vi "Nimbelink_Database_Ops_No_SQL_Open_Close.vi"(0 "Operation":T1(ring)=enum."Get Col Names", 1 "Find column":u16(ring) items=["work_order", "btw_sn", "mac", "meid", "operator", "datetime", "part_number", "imei", "sim_id", "phone", "test_result"], 2 "table name":string="test_data", 5 "Record data":string[](array[string])=["wo12345", "123450001", "70B3D55A8100", "A1001234567890", "Joe", "2013-05-07 10:28:19", "100013", "353123456789012", "89123456789012345678", "612-555-1212", "Pass", "", "", "", "", "", "", "", "", "", "", "", "", "", "", "", "", "", "", "", "", "", "", "", "", "", "", "", "", "", "", "", "", "", "", "", "", "", "", "", "", "", "", "", "", "", "", "", "", "", "", "", "12:01:00"], 7 "Connection In":refnum<k7>, 9 "SQL Query":string="Insert into dbo.test_data VALUES ", 11 "Error in (no error)":errorcluster, 12 "Find data":string, 13 "Insert fields":i32=23) -> (3 "Found?":bool, 4 "RecordSet":string[][](array[string]), 6 "Column Names":string[](array[string])=["work_order", "btw_sn", "mac", "meid", "operator", "date_time", "part_number", "imei", "sim_id", "phone_number", "test_result", "board_sn", "test_time", "test_program", "test_version", "extra1", "extra2", "guid", "extra3", "extra4", "extra5", "extra6", "extra7"], 8 "Connection Out":refnum<k7>, 10 "Records":i32, 14 "Last test passed?":bool, 15 "Error out":errorcluster)   [LabVIEW 2013]
panel:
  out "Find return string":string
  out "Final query string":string="select column_name,* from information_schema.columns\n where table_name = 'test_data'\norder by ordinal_position"
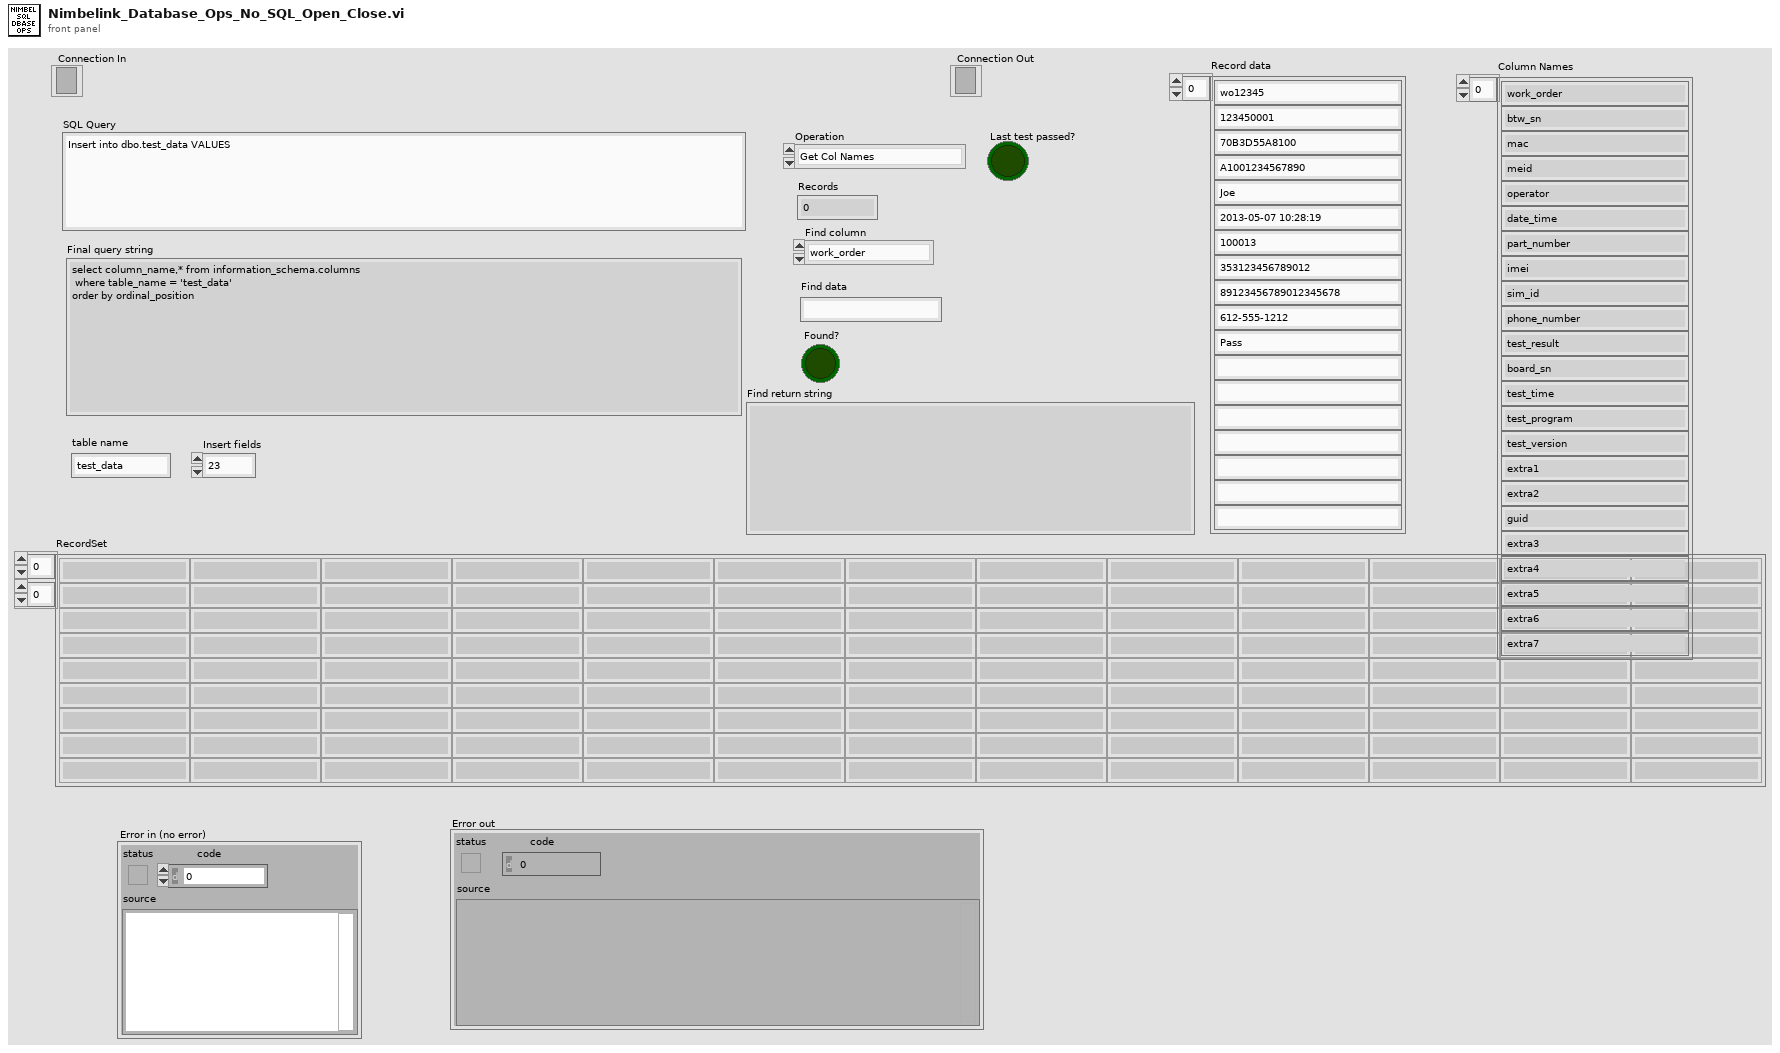
[diagram p1: front panel]
types:
  T1 = enum16{"Query", "Insert", "Select", "Dump Recs", "Get Rec Count", "Get Col Names", "Insert all fields", "Find", "Get last test result", "Get work order qty", "Set work order qty", "Save test report", "Get test report", "Execute query no data", "Select count", "Query and return row 0 col 0"}
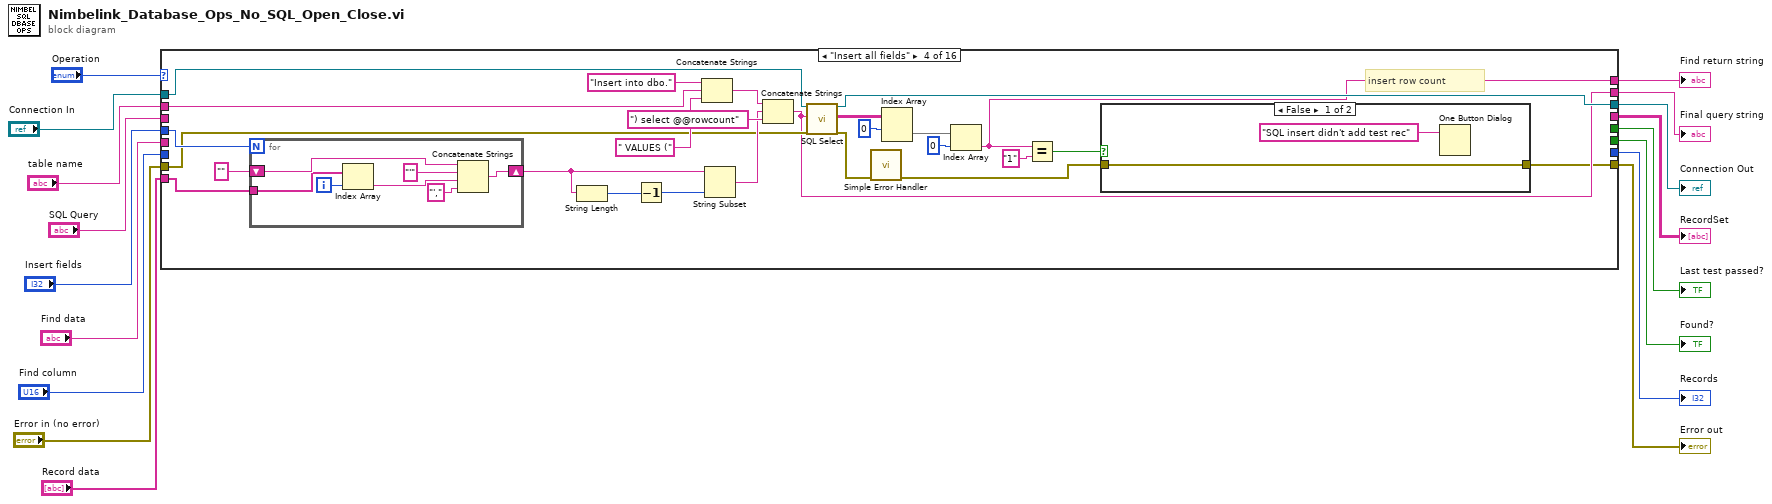
[diagram p0: block diagram]
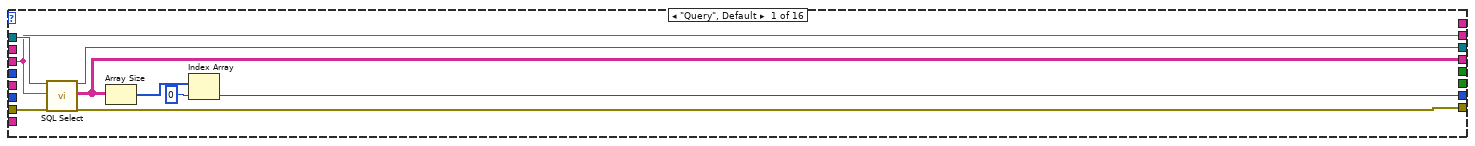
[diagram p2: hidden frame]
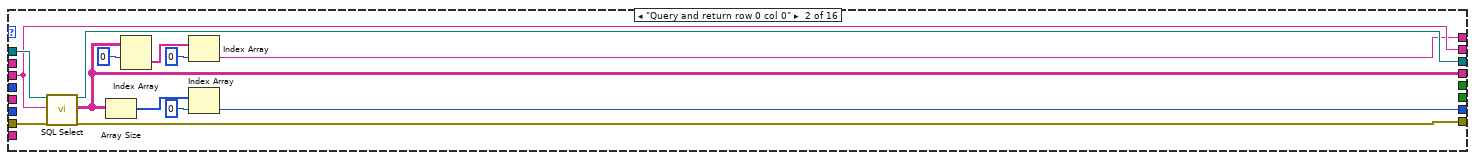
[diagram p3: hidden frame]
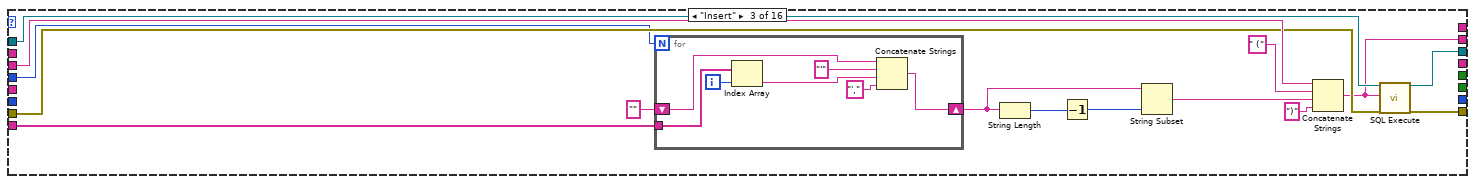
[diagram p4: hidden frame]
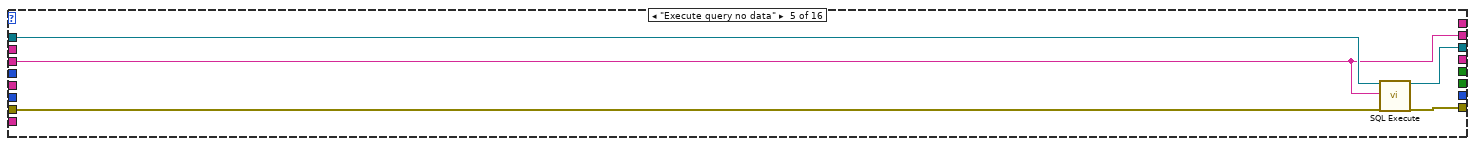
[diagram p6: hidden frame]
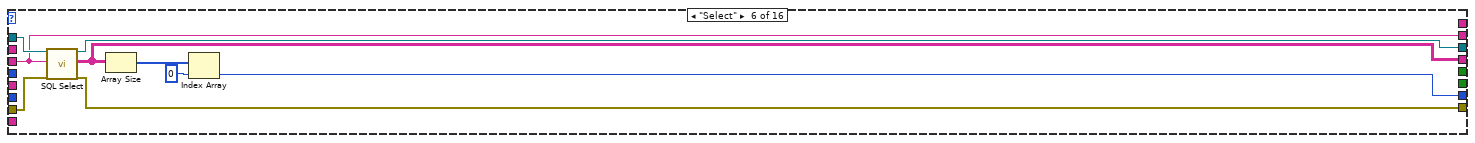
[diagram p7: hidden frame]
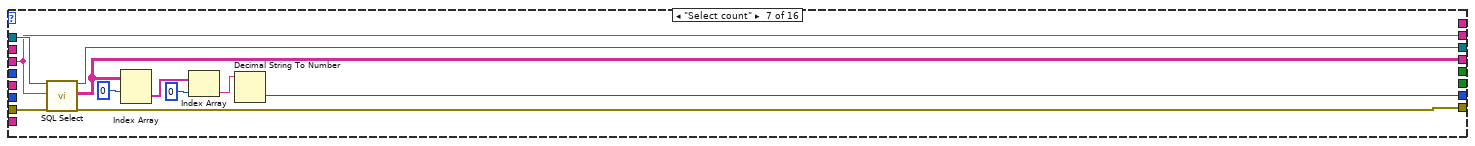
[diagram p8: hidden frame]
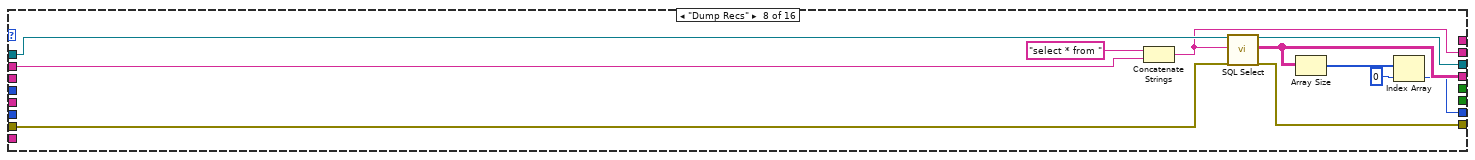
[diagram p9: hidden frame]
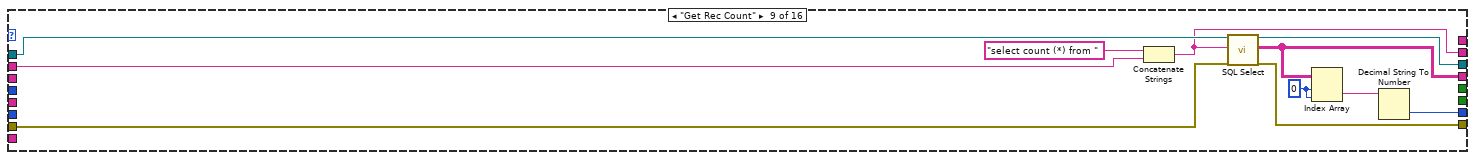
[diagram p10: hidden frame]
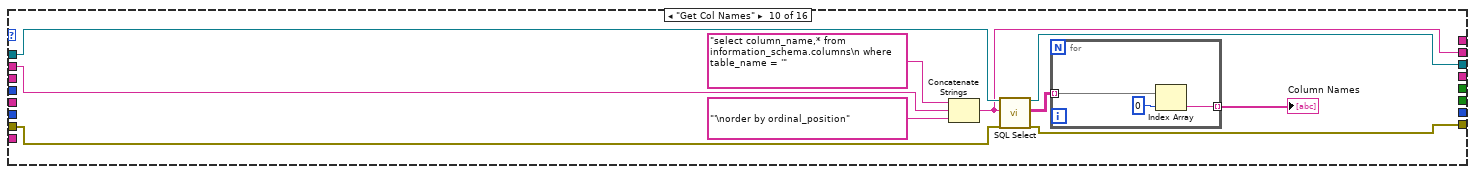
[diagram p11: hidden frame]
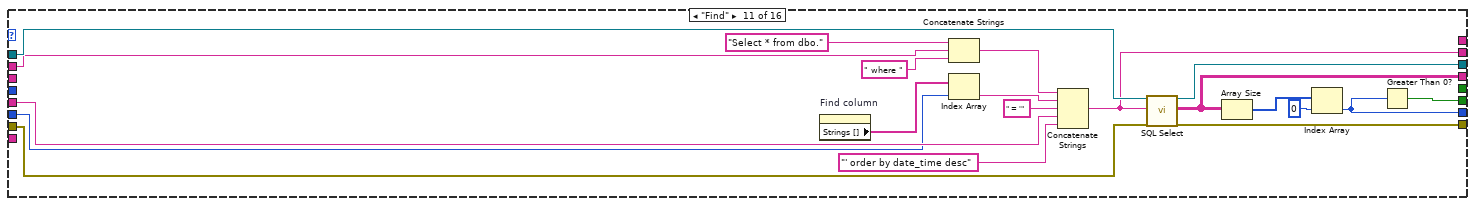
[diagram p12: hidden frame]
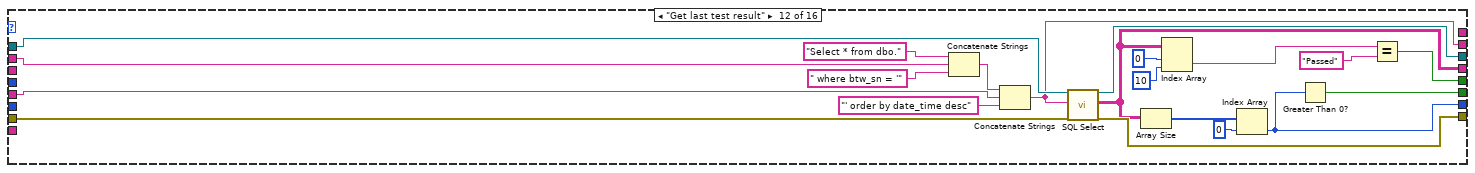
[diagram p13: hidden frame]
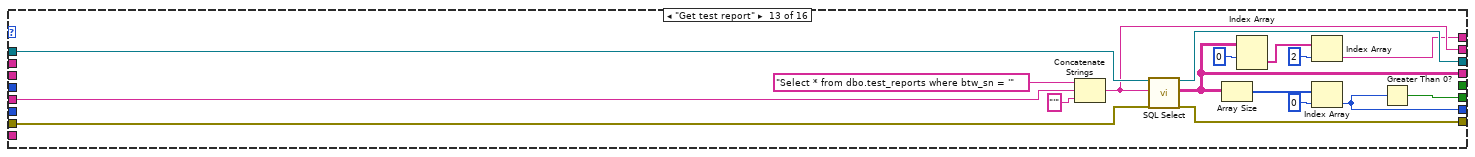
[diagram p14: hidden frame]
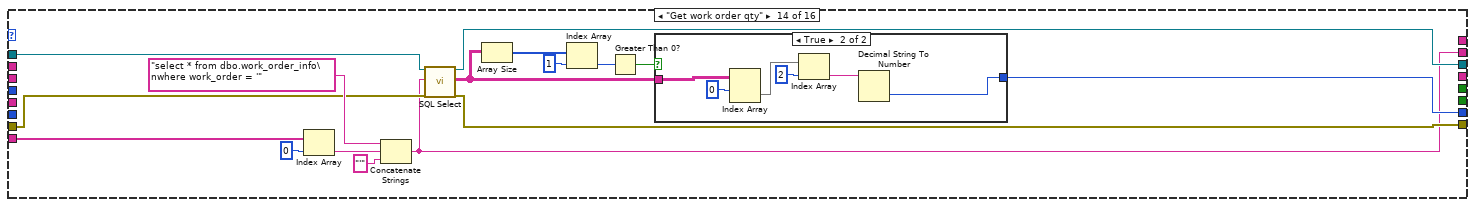
[diagram p15: hidden frame]
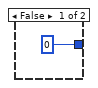
[diagram p16: hidden frame]
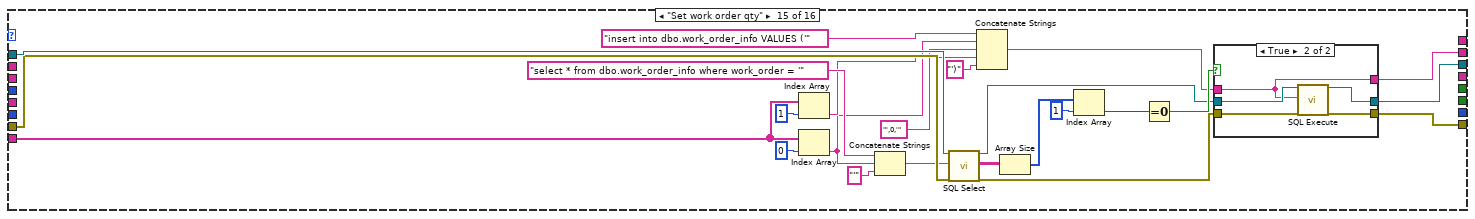
[diagram p17: hidden frame]
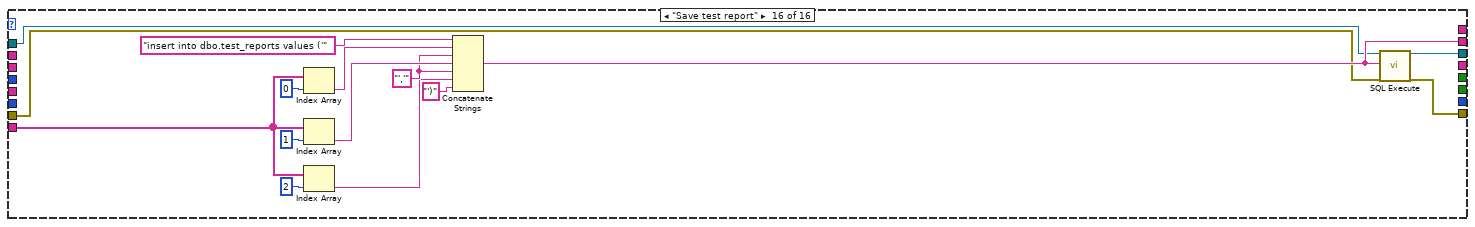
[diagram p19: hidden frame]
diagram:
  n1 = case shown="\"Insert all fields\"" "Operation" {
    tunnel: [w25 w38 w54 w62 w102 w108 w119 w130 w141 w150 w171 w195 w212 w220 w246 w280] -> w1
    tunnel: [w23 w36 w53 w74 w101 w109 w120 w131 w142 w149 w173 w197 w214 w222 w245 w279] -> w17
    tunnel: "Connection In" -> [w24 w37 w52 w75 w100 w110 w121 w133 w144 w154 w174 w198 w215 w223 w262 w276]
    tunnel: "Error in (no error)" -> [w26 w39 w42 w73 w99 w111 w122 w132 w143 w153 w172 w196 w213 w225 w259 w277]
    tunnel: "SQL Query" -> [w22 w35 w47 _ w98 w107 w118 _ _ _ _ _ _ _ _ _]
    tunnel: [w19 w31 _ _ _ w104 w117 w126 w136 _ w168 w183 w203 _ _ _] -> w12
    tunnel: "Record data" -> [_ _ w51 w87 _ _ _ _ _ _ _ _ _ w224 w251 w275]
    tunnel: [w22 w35 w41 w68 w98 w107 w118 w129 w138 w148 w167 w192 w209 w219 w244 w278] -> w13
    tunnel: "table name" -> [_ _ _ w80 _ _ _ w128 w139 w146 w164 w189 _ _ _ _]
    tunnel: [w18 w32 _ _ _ w103 w112 w123 w135 _ w161 w186 w207 w221 _ _] -> w10
    tunnel: [_ _ _ _ _ _ _ _ _ _ w160 w185 w206 _ _ _] -> w9
    tunnel: "Find data" -> [_ _ _ _ _ _ _ _ _ _ w159 w184 w205 _ _ _]
    tunnel: "Find column" -> [_ _ _ _ _ _ _ _ _ _ w158 _ _ _ _ _]
    tunnel: [_ _ _ _ _ _ _ _ _ _ _ w178 _ _ _ _] -> w6
    tunnel: "Insert fields" -> [_ _ w40 w76 _ _ _ _ _ _ _ _ _ _ _ _]
    tunnel: [_ w27 _ w66 _ _ _ _ _ _ _ _ w200 _ _ _] -> w4
    frame "Query", Default {
      n2 = call "SQL Select.vi"("Connection In"=w24, "SQL Query"=w22, "Error in (no error)"=w26) -> ("Connection Out"=w23:refnum<k7>, "Data"=w19:string[][], "Error out"=w25:errorcluster)  [unwired: 14 in]
      n3 = Array Size(array=w19) -> (size(s)=w21:i32[])
      n4 = Index Array(array=w21, index=0) -> (element=w18:i32)
    }
    frame "Query and return row 0 col 0" {
      n5 = call "SQL Select.vi"("Connection In"=w37, "SQL Query"=w35, "Error in (no error)"=w39) -> ("Connection Out"=w36:refnum<k7>, "Data"=w31:string[][], "Error out"=w38:errorcluster)  [unwired: 14 in]
      n6 = Array Size(array=w31) -> (size(s)=w34:i32[])
      n7 = Index Array(array=w31, index (row)=0) -> (element=w29:string[])  [unwired: 1 in]
      n8 = Index Array(array=w29, index=0) -> (element=w27:string)
      n9 = Index Array(array=w34, index=0) -> (element=w32:i32)
    }
    frame "Insert" {
      n10 = for {
        N: w40 -> [_]
        tunnel: w51 -> [w57]
        shift-right: [w60] -> w44
        shift-left: "" -> [w59]
        i -> [w56]
        n11 = Index Array(array=w57, index=w56) -> (element=w55:string)
        n12 = Concatenate Strings(w59, "'" ("string"), w55, "'," ("string")) -> (w60:string)
      }
      n13 = String Length(string=w44) -> (length=w46:i32)
      n14 = Decrement(x=w46) -> (x-1=w45:i32)
      n15 = String Subset(string=w44, length (rest)=w45) -> (substring=w43:string)  [unwired: 1 in]
      n16 = Concatenate Strings(w47, " (" ("string"), w43, ")") -> (w41:string)
      n17 = call "SQL Execute.vi"("Connection In"=w52, "SQL Query"=w41, "Error in (no error)"=w42) -> ("Connection Out"=w53:refnum<k7>, "Error out"=w54:errorcluster)  [unwired: 15 in]
    }
    frame "Insert all fields" {
      # "insert row count"
      n18 = for {
        N: w76 -> [_]
        tunnel: w87 -> [w93]
        shift-right: [w96] -> w82
        shift-left: "" -> [w95]
        i -> [w92]
        n19 = Index Array(array=w93, index=w92) -> (element=w91:string)
        n20 = Concatenate Strings(w95, "'" ("string"), w91, "'," ("string")) -> (w96:string)
      }
      n21 = String Length(string=w82) -> (length=w84:i32)
      n22 = Decrement(x=w84) -> (x-1=w83:i32)
      n23 = Concatenate Strings("Insert into dbo." ("string"), w80, " VALUES (" ("string")) -> (w79:string)
      n24 = String Subset(string=w82, length (rest)=w83) -> (substring=w81:string)  [unwired: 1 in]
      n25 = Concatenate Strings(w79, w81, ") select @@rowcount") -> (w68:string)
      n26 = call "SQL Select.vi"("Connection In"=w75, "SQL Query"=w68, "Error in (no error)"=w73) -> ("Connection Out"=w74:refnum<k7>, "Data"=w69:string[][], "Error out"=w67:errorcluster)  [unwired: 14 in]
      n27 = call <vilib>:"Simple Error Handler.vi"("error in (no error)"=w67) -> ("error out"=w63:errorcluster)  [unwired: 4 in, 4 out]
      n28 = Index Array(array=w69, index (row)=0) -> (element=w71:string[])  [unwired: 1 in]
      n29 = Index Array(array=w71, index=0) -> (element=w66:string)
      n30 = Equal?(x=w66, y="1") -> (x = y?=w64:bool)
      n31 = case shown="False" w64 {
        tunnel: w63 -> [w88 w90]
        tunnel: [w88 w90] -> w62
        frame False {
          n32 = One Button Dialog(message="SQL insert didn't add test rec") -> ()  [unwired: 1 in, 1 out]
        }
        frame True {
        }
      }
    }
    frame "Execute query no data" {
      n33 = call "SQL Execute.vi"("Connection In"=w100, "SQL Query"=w98, "Error in (no error)"=w99) -> ("Connection Out"=w101:refnum<k7>, "Error out"=w102:errorcluster)  [unwired: 15 in]
    }
    frame "Select" {
      n34 = call "SQL Select.vi"("Connection In"=w110, "SQL Query"=w107, "Error in (no error)"=w111) -> ("Connection Out"=w109:refnum<k7>, "Data"=w104:string[][], "Error out"=w108:errorcluster)  [unwired: 14 in]
      n35 = Array Size(array=w104) -> (size(s)=w106:i32[])
      n36 = Index Array(array=w106, index=0) -> (element=w103:i32)
    }
    frame "Select count" {
      n37 = call "SQL Select.vi"("Connection In"=w121, "SQL Query"=w118, "Error in (no error)"=w122) -> ("Connection Out"=w120:refnum<k7>, "Data"=w117:string[][], "Error out"=w119:errorcluster)  [unwired: 14 in]
      n38 = Index Array(array=w117, index (row)=0) -> (element=w115:string[])  [unwired: 1 in]
      n39 = Index Array(array=w115, index=0) -> (element=w113:string)
      n40 = Decimal String To Number(string=w113) -> (number=w112:i32)  [unwired: 2 in, 1 out]
    }
    frame "Dump Recs" {
      n41 = Concatenate Strings("select * from " ("SQL Query"), w128) -> (w129:string)
      n42 = call "SQL Select.vi"("Connection In"=w133, "SQL Query"=w129, "Error in (no error)"=w132) -> ("Connection Out"=w131:refnum<k7>, "Data"=w126:string[][], "Error out"=w130:errorcluster)  [unwired: 14 in]
      n43 = Array Size(array=w126) -> (size(s)=w125:i32[])
      n44 = Index Array(array=w125, index=0) -> (element=w123:i32)
    }
    frame "Get Rec Count" {
      w140 = 0 ("index (row)")
      n45 = Concatenate Strings("select count (*) from " ("SQL Query"), w139) -> (w138:string)
      n46 = call "SQL Select.vi"("Connection In"=w144, "SQL Query"=w138, "Error in (no error)"=w143) -> ("Connection Out"=w142:refnum<k7>, "Data"=w136:string[][], "Error out"=w141:errorcluster)  [unwired: 14 in]
      n47 = Index Array(array=w136, index (row)=w140, index (col)=w140) -> (element=w134:string)
      n48 = Decimal String To Number(string=w134) -> (number=w135:i32)  [unwired: 2 in, 1 out]
    }
    frame "Get Col Names" {
      n49 = Concatenate Strings("select column_name,* from information_schema.columns\n where table_name = '" ("SQL Query"), w146, "'\norder by ordinal_position" ("SQL Query")) -> (w148:string)
      n50 = call "SQL Select.vi"("Connection In"=w154, "SQL Query"=w148, "Error in (no error)"=w153) -> ("Connection Out"=w149:refnum<k7>, "Data"=w152:string[][], "Error out"=w150:errorcluster)  [unwired: 14 in]
      n51 = for {
        tunnel: w152 -> [w157] mode=indexing
        tunnel: [w156] -> w151 mode=indexing
        n52 = Index Array(array=w157, index=0 ("index (col)")) -> (element=w156:string)
      }
      "Column Names" <- w151
    }
    frame "Find" {
      n53 = property on="Find column" class="Ring (strict)"() -> ("Strings []"=w177:string[])  [unwired: 2 in, 2 out]
      n54 = Concatenate Strings("Select * from dbo." ("string"), w164, " where " ("string")) -> (w166:string)
      n55 = Index Array(array=w177, index=w158) -> (element=w176:string)
      n56 = Concatenate Strings(w166, w176, " = '" ("string"), w159, "' order by date_time desc" ("string")) -> (w167:string)
      n57 = call "SQL Select.vi"("Connection In"=w174, "SQL Query"=w167, "Error in (no error)"=w172) -> ("Connection Out"=w173:refnum<k7>, "Data"=w168:string[][], "Error out"=w171:errorcluster)  [unwired: 14 in]
      n58 = Array Size(array=w168) -> (size(s)=w169:i32[])
      n59 = Index Array(array=w169, index=0) -> (element=w161:i32)
      n60 = Greater Than 0?(x=w161) -> (x > 0?=w160:bool)
    }
    frame "Get last test result" {
      n61 = Concatenate Strings("Select * from dbo." ("string"), w189, " where btw_sn = '" ("string")) -> (w191:string)
      n62 = Concatenate Strings(w191, w184, "' order by date_time desc" ("string")) -> (w192:string)
      n63 = call "SQL Select.vi"("Connection In"=w198, "SQL Query"=w192, "Error in (no error)"=w196) -> ("Connection Out"=w197:refnum<k7>, "Data"=w183:string[][], "Error out"=w195:errorcluster)  [unwired: 14 in]
      n64 = Array Size(array=w183) -> (size(s)=w193:i32[])
      n65 = Index Array(array=w183, index (row)=0, index (col)=10 ("disabled index (col)")) -> (element=w180:string)
      n66 = Index Array(array=w193, index=0) -> (element=w186:i32)
      n67 = Greater Than 0?(x=w186) -> (x > 0?=w185:bool)
      n68 = Equal?(x=w180, y="Passed") -> (x = y?=w178:bool)
    }
    frame "Get test report" {
      n69 = Concatenate Strings("Select * from dbo.test_reports where btw_sn = '" ("string"), w205, "'" ("string")) -> (w209:string)
      n70 = call "SQL Select.vi"("Connection In"=w215, "SQL Query"=w209, "Error in (no error)"=w213) -> ("Connection Out"=w214:refnum<k7>, "Data"=w203:string[][], "Error out"=w212:errorcluster)  [unwired: 14 in]
      n71 = Array Size(array=w203) -> (size(s)=w210:i32[])
      n72 = Index Array(array=w203, index (row)=0) -> (element=w201:string[])  [unwired: 1 in]
      n73 = Index Array(array=w201, index=2) -> (element=w200:string)
      n74 = Index Array(array=w210, index=0) -> (element=w207:i32)
      n75 = Greater Than 0?(x=w207) -> (x > 0?=w206:bool)
    }
    frame "Get work order qty" {
      n76 = Index Array(array=w224, index=0) -> (element=w227:string)
      n77 = Concatenate Strings("select * from dbo.work_order_info\nwhere work_order = '" ("SQL Query"), w227, "'" ("string")) -> (w219:string)
      n78 = call "SQL Select.vi"("Connection In"=w223, "SQL Query"=w219, "Error in (no error)"=w225) -> ("Connection Out"=w222:refnum<k7>, "Data"=w218:string[][], "Error out"=w220:errorcluster)  [unwired: 14 in]
      n79 = Array Size(array=w218) -> (size(s)=w217:i32[])
      n80 = Index Array(array=w217, index=1) -> (element=w216:i32)
      n81 = Greater Than 0?(x=w216) -> (x > 0?=w226:bool)
      n82 = case shown="True" w226 {
        tunnel: w218 -> [_ w237]
        tunnel: [0 w236] -> w221
        frame False {
        }
        frame True {
          n83 = Index Array(array=w237, index (row)=0 ("index")) -> (element=w235:string[])  [unwired: 1 in]
          n84 = Index Array(array=w235, index=2) -> (element=w233:string)
          n85 = Decimal String To Number(string=w233) -> (number=w236:i32)  [unwired: 2 in, 1 out]
        }
      }
    }
    frame "Set work order qty" {
      n86 = Index Array(array=w251, index=1) -> (element=w252:string)
      n87 = Index Array(array=w251, index=0) -> (element=w250:string)
      n88 = Concatenate Strings("select * from dbo.work_order_info where work_order = '" ("SQL Query"), w250, "'" ("string")) -> (w243:string)
      n89 = call "SQL Select.vi"("Connection In"=w262, "SQL Query"=w243, "Error in (no error)"=w259) -> ("Connection Out"=w248:refnum<k7>, "Data"=w239:string[][], "Error out"=w247:errorcluster)  [unwired: 14 in]
      n90 = Concatenate Strings("insert into dbo.work_order_info VALUES ('" ("SQL Query"), w250, "',0,'" ("string"), w252, "')" ("string")) -> (w240:string)
      n91 = Array Size(array=w239) -> (size(s)=w242:i32[])
      n92 = Index Array(array=w242, index=1) -> (element=w241:i32)
      n93 = Equal To 0?(x=w241) -> (x = 0?=w257:bool)
      n94 = case shown="True" w257 {
        tunnel: w248 -> [w264 w267]
        tunnel: w240 -> [w263 w266]
        tunnel: w247 -> [w265 w270]
        tunnel: [w265 w269] -> w246
        tunnel: [w264 w268] -> w245
        tunnel: [w263 w266] -> w244
        frame False {
        }
        frame True {
          n95 = call "SQL Execute.vi"("Connection In"=w267, "SQL Query"=w266, "Error in (no error)"=w270) -> ("Connection Out"=w268:refnum<k7>, "Error out"=w269:errorcluster)  [unwired: 15 in]
        }
      }
    }
    frame "Save test report" {
      w273 = "','" ("string")
      n96 = Index Array(array=w275, index=0) -> (element=w281:string)
      n97 = Index Array(array=w275, index=1) -> (element=w282:string)
      n98 = Index Array(array=w275, index=2) -> (element=w272:string)
      n99 = Concatenate Strings("insert into dbo.test_reports values ('" ("SQL Query"), w281, w273, w282, w273, w272, "')" ("string")) -> (w278:string)
      n100 = call "SQL Execute.vi"("Connection In"=w276, "SQL Query"=w278, "Error in (no error)"=w277) -> ("Connection Out"=w279:refnum<k7>, "Error out"=w280:errorcluster)  [unwired: 15 in]
    }
  }
  "Error out" <- w1
  "RecordSet" <- w12
  "Final query string" <- w13
  "Records" <- w10
  "Found?" <- w9
  "Last test passed?" <- w6
  "Find return string" <- w4
  "Connection Out" <- w17
